vi "Test_Settings_Call_FGV.vi"() -> ()   [LabVIEW 2015]
uses:
  controls/EXPERIMENT_Inputs.ctl
  controls/LASER_Inputs.ctl
  controls/SOFTWARE_Inputs.ctl
  controls/AO_6711_Inputs.ctl
  <instrlib>/niHSDIO/niHSDIO.llb/niHSDIO_ctl Trigger Source Values (Ring).ctl
  controls/HSDIO_6541_Inputs.ctl
  controls/AWG_5421_Inputs.ctl
  <instrlib>/niScope/Controls/niScope trigger source.ctl
  controls/DIGIT_5122_Inputs.ctl
  controls/HARDWARE_Inputs.ctl
  <instrlib>/niFgen/niFgen.llb/niFgen_ctl Trigger Source Values (Ring).ctl
  controls/TRAPPING_Inputs.ctl
panel:
  in  "HARDWARE Inputs":T1={"AO 6711 Inputs"={"Physical Channels"="AnalogOutput/ao0:3", "Min Voltage"=-10.0, "Max Voltage"=10.0, "Trigger Source"="/AnalogOutput/PFI0", "counter"="AnalogOutput/ctr0"}, "AWG 5421 Inputs"={"Resource Name"="WaveformGenerator", "Sample Rate"=20000000.0, "Trigger Type"=2, "Trigger Source"="PFI0", "Waveform Gain"=0.31, "Digital Filter ON"=TRUE}, "DIGIT 5122 Inputs"={"Sample Rate"=10000000.0, "Resource Name"="Digitizer", "Channel Name"="0", "Trigger Source"="VAL_EXTERNAL", "Vertical Range"=10.0, "Trigger Level"=3.0}, "HSDIO 6541 Inputs"={"Resource Name"="SequencerHSDIO", "Clock Rate"=1000000.0, "Trigger Source"="PFI0"}} {"HSDIO 6541 Inputs"."Clock Rate" format="%.2p"; "DIGIT 5122 Inputs"."Trigger Level" format="%.2f"; "DIGIT 5122 Inputs"."Vertical Range" format="%.2f"; "DIGIT 5122 Inputs"."Sample Rate" step=65535.0 format="%#_3p"; "AWG 5421 Inputs"."Sample Rate" format="%.2p"; "AWG 5421 Inputs"."Trigger Type" items=["None", "Software Edge", "Digital Edge", "Digital Level"]; "AO 6711 Inputs"."Max Voltage" min=-10.0 max=10.0; "AO 6711 Inputs"."Min Voltage" min=-10.0 max=10.0}
  in  "EXPERIMENT Inputs":T9={"Date"="", "User Name"="", "Comment"="", "Experiment Steps"=[], "Sample Components"=[], "Molecules"=[], "Laser 1"={"Used"=TRUE, "Name"="Spectroscopy", "Reference"="Yag", "Wavelength"=1000.0, "Energy"=25.0}, "Laser 2"={"Used"=TRUE, "Name"="Spectroscopy", "Reference"="Yag", "Wavelength"=1000.0, "Energy"=25.0}, "Laser 3"={"Used"=TRUE, "Name"="Spectroscopy", "Reference"="Yag", "Wavelength"=1000.0, "Energy"=25.0}}
  in  "SOFTWARE Inputs":T11={"Application Directory"=path "D:/PIRENEA/DATA", "Resources Path"=path "D:/S.O.F.T.S/LABVIEW/PIL/resources", "Data Path"=path "D:/PIRENEA/DATA", "XML Path"=path "D:/PIRENEA/DATA", "XML File Filter"="/AnalogOutput/PFI0", "Excit Scripts Path"=path "D:/PIRENEA/EXCIT_SCRIPTS", "Excit Scripts File Filter"="*.txt", "Excit Waveforms Path"=path "D:/PIRENEA/EXCIT_WFMS", "Excit Waveforms File Filter"="*.bin", "Timing Scripts Path"=path "D:/PIRENEA/SEQUENCE_SCRIPTS", "Timing Scripts File Filter"="*.txt", "Timing Waveforms Path"=path "D:/PIRENEA/SEQUENCE_WFMS", "Timing Waveforms File Filter"="*.bin", "Trapping Waveforms Path"=path "D:/PIRENEA/TRAPPING_WFMS", "Trapping Waveforms File Filter"="*.bin"}
  in  "TRAPPING Inputs":T12={"Number of Channels"=4, "Init Values"=[2.0, 9.0, 2.0, 9.0], "Opening Values"=[0.0, 0.0, 0.0, 0.0], "Trapping Values"=[2.0, 9.0, 2.0, 9.0], "Emptying Values"=[-10.0, -10.0, -10.0, -10.0], "Adiabatic ON"=FALSE, "Adiabatic Duration"=100, "Adiabatic Waveforms"=["Adiabatic_None_2_2_2000", "Adiabatic_Ramp_9_0_2000", "Adiabatic_None_2_2_2000", "Adiabatic_RC_9_0_2000"]} {"Trapping Values" min=-10.0 max=10.0; "Init Values" min=-10.0 max=10.0; "Emptying Values" min=-10.0 max=10.0; "Opening Values" min=-10.0 max=10.0}
  out "error out":errorcluster
  in  "error in (no error)":errorcluster caption="entrée d'erreur (pas d'erreur)"
  # "Name"
  # "Reference"
  # "(nm)"
  # "E (J)"
  # "Laser 1"
  # "Laser 2"
  # "Laser 3"
  # "GO_out"
  # "Gout"
  # "GI_in"
  # "Gin"
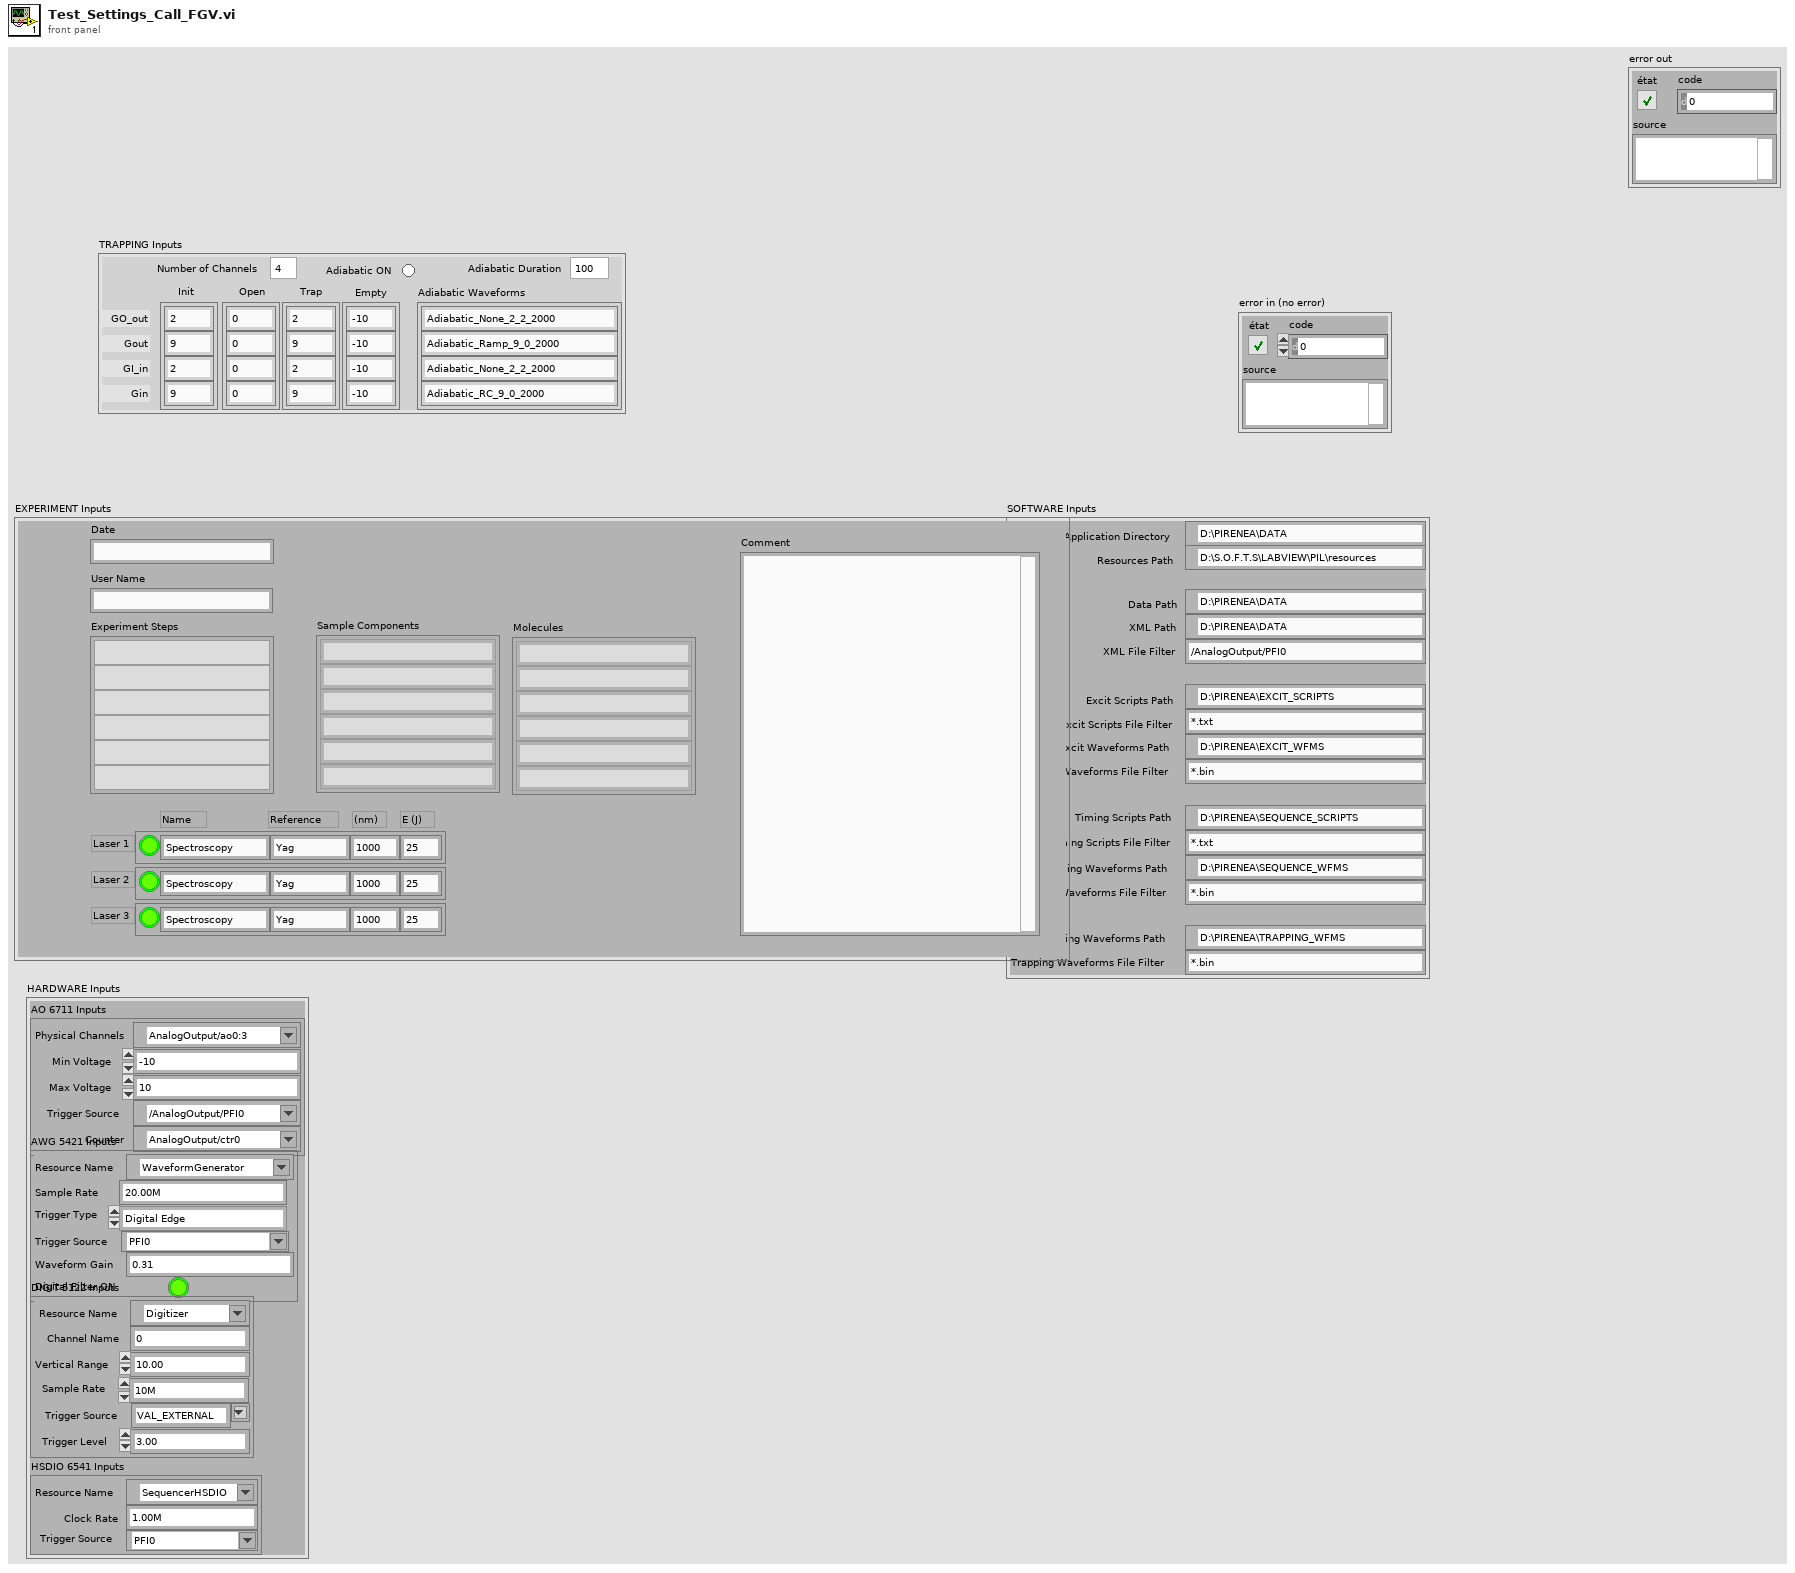
[diagram p1: front panel]
types:
  T1 = typedef "HARDWARE_Inputs.ctl" = cluster{"AO 6711 Inputs":T2, "AWG 5421 Inputs":T3, "DIGIT 5122 Inputs":T5, "HSDIO 6541 Inputs":T7}
  T2 = typedef "AO_6711_Inputs.ctl" = cluster{"Physical Channels":tag, "Min Voltage":dbl, "Max Voltage":dbl, "Trigger Source":tag, "counter":tag}
  T3 = typedef "AWG_5421_Inputs.ctl" = cluster{"Resource Name":refnum<k15>, "Sample Rate":dbl, "Trigger Type":u16, "Trigger Source":T4, "Waveform Gain":dbl, "Digital Filter ON":bool}
  T4 = typedef "niFgen_ctl Trigger Source Values (Ring).ctl" = string
  T5 = typedef "DIGIT_5122_Inputs.ctl" = cluster{"Sample Rate":dbl, "Resource Name":refnum<k15>, "Channel Name":string, "Trigger Source":T6, "Vertical Range":dbl, "Trigger Level":dbl}
  T6 = typedef "niScope trigger source.ctl" = string
  T7 = typedef "HSDIO_6541_Inputs.ctl" = cluster{"Resource Name":refnum<k15>, "Clock Rate":dbl, "Trigger Source":T8}
  T8 = typedef "niHSDIO_ctl Trigger Source Values (Ring).ctl" = string
  T9 = typedef "EXPERIMENT_Inputs.ctl" = cluster{"Date":string, "User Name":string, "Comment":string, "Experiment Steps":string[], "Sample Components":string[], "Molecules":string[], "Laser 1":T10, "Laser 2":T10, "Laser 3":T10}
  T10 = typedef "LASER_Inputs.ctl" = cluster{"Used":bool, "Name":string, "Reference":string, "Wavelength":dbl, "Energy":dbl}
  T11 = typedef "SOFTWARE_Inputs.ctl" = cluster{"Application Directory":path, "Resources Path":path, "Data Path":path, "XML Path":path, "XML File Filter":string, "Excit Scripts Path":path, "Excit Scripts File Filter":string, "Excit Waveforms Path":path, "Excit Waveforms File Filter":string, "Timing Scripts Path":path, "Timing Scripts File Filter":string, "Timing Waveforms Path":path, "Timing Waveforms File Filter":string, "Trapping Waveforms Path":path, "Trapping Waveforms File Filter":string}
  T12 = typedef "TRAPPING_Inputs.ctl" = cluster{"Number of Channels":i32, "Init Values":dbl[], "Opening Values":dbl[], "Trapping Values":dbl[], "Emptying Values":dbl[], "Adiabatic ON":bool, "Adiabatic Duration":i32, "Adiabatic Waveforms":string[]}
  T13 = enum16{"Set", "Get", "Read XML", "Write XML", "Convert to String"}
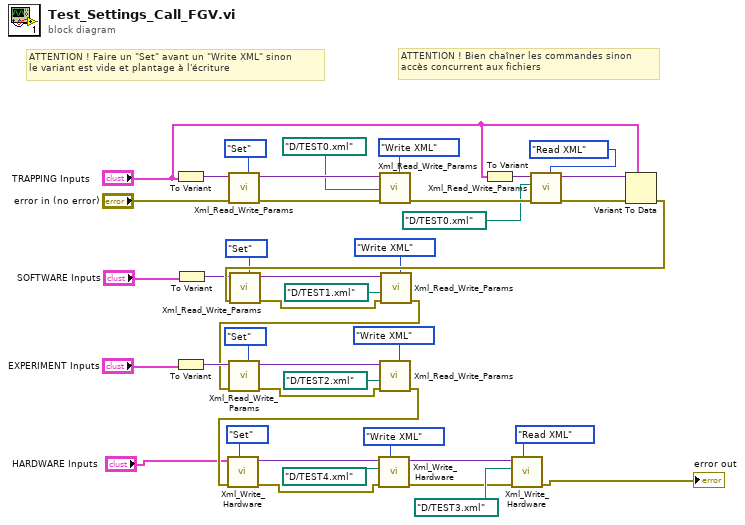
[diagram p0: block diagram]
diagram:
  # "ATTENTION ! Bien chaîner les commandes sinon\naccès concurrent aux fichiers"
  # "ATTENTION ! Faire un \"Set\" avant un \"Write XML\" sinon\nle variant est vide et plantage à l'écriture"
  n1 = To Variant(anything="TRAPPING Inputs") -> (Variant=w32:variant)
  n2 = To Variant(anything="EXPERIMENT Inputs") -> (Variant=w8:variant)
  n3 = To Variant(anything="SOFTWARE Inputs") -> (Variant=w15:variant)
  n4 = call "Xml_Read_Write_Params.vi"("Variant"=w32, "error in (no error)"="error in (no error)", "Command"=enum16{"Read XML", "Set", "Get", "Write XML"}."Set") -> ("Variant Output"=w30:variant, "error out"=w29:errorcluster)  [unwired: 4 in, 1 out]
  n5 = call "Xml_Read_Write_Params.vi"("Variant"=w30, "XML Path"=path "D:/TEST0.xml", "error in (no error)"=w29, "Command"=enum16{"Read XML", "Set", "Get", "Write XML"}."Write XML") -> ("error out"=w27:errorcluster)  [unwired: 3 in, 2 out]
  n6 = To Variant(anything="TRAPPING Inputs") -> (Variant=w20:variant)
  n7 = call "Xml_Read_Write_Params.vi"("Variant"=w20, "XML Path"=path "D:/TEST0.xml", "error in (no error)"=w27, "Command"=enum16{"Read XML", "Set", "Get", "Write XML"}."Read XML") -> ("Variant Output"=w24:variant, "error out"=w23:errorcluster)  [unwired: 3 in, 1 out]
  n8 = Variant To Data(error in=w23, type="TRAPPING Inputs", Variant=w24) -> (error out=w22:errorcluster)  [unwired: 1 out]
  n9 = call "Xml_Read_Write_Params.vi"("Variant"=w15, "error in (no error)"=w22, "Command"=enum16{"Read XML", "Set", "Get", "Write XML"}."Set") -> ("Variant Output"=w17:variant, "error out"=w18:errorcluster)  [unwired: 4 in, 1 out]
  n10 = call "Xml_Read_Write_Params.vi"("Variant"=w17, "XML Path"=path "D:/TEST1.xml", "error in (no error)"=w18, "Command"=enum16{"Read XML", "Set", "Get", "Write XML"}."Write XML") -> ("error out"=w4:errorcluster)  [unwired: 3 in, 2 out]
  n11 = call "Xml_Read_Write_Params.vi"("Variant"=w8, "error in (no error)"=w4, "Command"=enum16{"Read XML", "Set", "Get", "Write XML"}."Set") -> ("Variant Output"=w6:variant, "error out"=w5:errorcluster)  [unwired: 4 in, 1 out]
  n12 = call "Xml_Read_Write_Params.vi"("Variant"=w6, "XML Path"=path "D:/TEST2.xml", "error in (no error)"=w5, "Command"=enum16{"Read XML", "Set", "Get", "Write XML"}."Write XML") -> ("error out"=w40:errorcluster)  [unwired: 3 in, 2 out]
  n13 = call "Xml_Write_Hardware.vi"(7:T13."Set" ("Command"), "error in (no error)"=w40, "Variant"="HARDWARE Inputs") -> ("error out"=w42:errorcluster, "Variant Output"=w38:variant)  [unwired: 6 in, 1 out]
  n14 = call "Xml_Write_Hardware.vi"(7:T13."Write XML" ("Command"), "error in (no error)"=w42, 10:path "D:/TEST4.xml" ("XML Path"), "Variant"=w38) -> ("error out"=w35:errorcluster, "Variant Output"=w37:variant)  [unwired: 5 in, 1 out]
  n15 = call "Xml_Write_Hardware.vi"(7:T13."Read XML" ("Command"), "error in (no error)"=w35, 10:path "D:/TEST3.xml" ("XML Path"), "Variant"=w37) -> ("error out"=→"error out":errorcluster)  [unwired: 5 in, 2 out]
